vi "read numarray, compare with original one.vi"(0 "JSON in":string, 1 "binary data in":u8[](array[numeric]), 5 "array as variant in":variant, 7 "numeric type":T1, 9 "kwarg_name":string, 11 "error in (no error)":errorcluster, 12 "dims":u8) -> (2 "current timepoint":dbl, 3 "numarray 1D":cdb[](array[numeric]), 4 "numarray 2D":cdb[][](array[numeric]), 6 "numarray 3D":cdb[][][](array[numeric]), 8 "type out":dbl, 10 "arrays are equal":bool, 13 "delta t (s)":dbl, 15 "error out":errorcluster)   [LabVIEW 2018, in "LV2Julia_core.lvlib"]
uses:
  LV2Julia_core.lvlib
  Numeric Types enum.ctl
  f90f2f60-c893-4d73-9894-bda48d86c5b6.vi
  1bcb8ed7-17cb-4152-8e47-ff7461b55bf4.vi
  05796eaf-ec06-43a6-a453-a404cbedcfeb.vi
  9b93abbe-6376-4f86-9348-90245d6e1835.vi
  760e0b37-cac3-4b4c-a236-19af47651068.vi
  729fa7d7-fd6d-49c0-b1c8-f0a08cd6f943.vi
  3b835e31-b93c-4e4c-9ac3-413a3184b071.vi
  5ec570e5-464f-4fa0-a09b-d89833ec3b5d.vi
  e2ab0a43-58c4-4b3b-8f56-301dfe696cbe.vi
  7bf60a27-5564-4d89-912b-dc8cfc55a1e3.vi
  6c204d97-3017-4fe4-991a-9f71cab6a49b.vi
  a9a31f31-ba5d-4a99-a09b-6ec61be075e6.vi
  2bab1b1a-04a3-4102-80c6-0860ef51feeb.vi
  f90f2f60-c893-4d73-9894-bda48d86c5b6.vi/32d88ae3-2c92-48bd-897b-7dd0343570a7.vi
  f90f2f60-c893-4d73-9894-bda48d86c5b6.vi/c53afe73-fc52-444d-a3d7-7d50831e1209.vi
  f90f2f60-c893-4d73-9894-bda48d86c5b6.vi/a66dcc77-dec5-41f4-a21e-acddf706e10f.vi
  f90f2f60-c893-4d73-9894-bda48d86c5b6.vi/4ba7e992-ac92-4a49-a2e7-98c2637664ea.vi
  1bcb8ed7-17cb-4152-8e47-ff7461b55bf4.vi/43da8a50-dff1-4339-a1c3-934883bf3cfa.vi
  1bcb8ed7-17cb-4152-8e47-ff7461b55bf4.vi/d0f3aec3-e539-46ad-9ed6-51bc67961256.vi
  1bcb8ed7-17cb-4152-8e47-ff7461b55bf4.vi/9e853403-19d2-43d7-8698-e40b975fe7e1.vi
  1bcb8ed7-17cb-4152-8e47-ff7461b55bf4.vi/e786b37f-7961-4d73-906c-7eb43609efd0.vi
  05796eaf-ec06-43a6-a453-a404cbedcfeb.vi/e1d72838-30cd-489b-8a44-cd7fcf5818b4.vi
  05796eaf-ec06-43a6-a453-a404cbedcfeb.vi/17980820-88c9-4418-a022-c645ed7312dc.vi
  05796eaf-ec06-43a6-a453-a404cbedcfeb.vi/41ee7d88-6397-4a7e-920a-8c7af2978bc3.vi
  05796eaf-ec06-43a6-a453-a404cbedcfeb.vi/82dbf2c0-5480-4f2b-a01b-b6af73a511fc.vi
  9b93abbe-6376-4f86-9348-90245d6e1835.vi/4ad5f33a-0790-406d-bfe1-08bba8267a66.vi
  9b93abbe-6376-4f86-9348-90245d6e1835.vi/c16bd300-9a14-44dd-a8e2-ac449f43e7b5.vi
  9b93abbe-6376-4f86-9348-90245d6e1835.vi/a0511438-dd98-4a92-986f-621a9f363a6a.vi
  9b93abbe-6376-4f86-9348-90245d6e1835.vi/c651fa37-4a64-4550-919d-369354992084.vi
  760e0b37-cac3-4b4c-a236-19af47651068.vi/09310928-e73b-456e-a29f-2af550aeed02.vi
  760e0b37-cac3-4b4c-a236-19af47651068.vi/082161be-e65e-418d-b5c3-addb765fb303.vi
  760e0b37-cac3-4b4c-a236-19af47651068.vi/948893fb-24fe-4050-867c-ffeb5abdf6bc.vi
  760e0b37-cac3-4b4c-a236-19af47651068.vi/9bc4b464-3baf-47a8-acda-6a3046ee8e10.vi
  729fa7d7-fd6d-49c0-b1c8-f0a08cd6f943.vi/4dc461b2-c442-4aea-8fe2-f79e850e50b6.vi
  729fa7d7-fd6d-49c0-b1c8-f0a08cd6f943.vi/f3471e8a-deba-4189-9c10-aa71fc9210b9.vi
  729fa7d7-fd6d-49c0-b1c8-f0a08cd6f943.vi/32030ce2-dff6-4f01-95b7-0827d636a462.vi
  729fa7d7-fd6d-49c0-b1c8-f0a08cd6f943.vi/c713e3f1-cad3-46f2-84b7-66f09a7e94ff.vi
  3b835e31-b93c-4e4c-9ac3-413a3184b071.vi/28cea966-c3ee-4471-b26a-6f175bc131ac.vi
  3b835e31-b93c-4e4c-9ac3-413a3184b071.vi/de96e9b0-be66-4c9e-9efc-c1f704469a1d.vi
  3b835e31-b93c-4e4c-9ac3-413a3184b071.vi/c00be31e-9a51-4a5a-83a6-45b490b9e683.vi
  3b835e31-b93c-4e4c-9ac3-413a3184b071.vi/ac6c025d-f474-4280-83b8-e9f6b8e68690.vi
  5ec570e5-464f-4fa0-a09b-d89833ec3b5d.vi/ca82bea4-4b91-4f8b-9f61-83a2a5577914.vi
  5ec570e5-464f-4fa0-a09b-d89833ec3b5d.vi/c4c3de46-0252-44a8-9010-5f8eb92ca105.vi
  5ec570e5-464f-4fa0-a09b-d89833ec3b5d.vi/e4886903-d285-4e62-8f40-eb3ebe842de4.vi
  5ec570e5-464f-4fa0-a09b-d89833ec3b5d.vi/fb6f816f-daa7-4e23-ba72-f885aa13bf06.vi
  e2ab0a43-58c4-4b3b-8f56-301dfe696cbe.vi/4e651908-bd94-4c47-b669-930f4933d222.vi
  e2ab0a43-58c4-4b3b-8f56-301dfe696cbe.vi/36ea2579-6193-4f32-b3f5-d90bd214050e.vi
  e2ab0a43-58c4-4b3b-8f56-301dfe696cbe.vi/95d4ced7-8003-4378-85ae-3062075d27bb.vi
  e2ab0a43-58c4-4b3b-8f56-301dfe696cbe.vi/454c1be2-9309-4afe-9153-ec44cf4b9f7f.vi
  7bf60a27-5564-4d89-912b-dc8cfc55a1e3.vi/8069382f-b1d8-4b8c-8509-eebfa9e45f70.vi
  7bf60a27-5564-4d89-912b-dc8cfc55a1e3.vi/5c067dbe-246b-42e9-9137-861b00fe523e.vi
  7bf60a27-5564-4d89-912b-dc8cfc55a1e3.vi/03b17b19-1ffb-46cc-8dc1-1c496a915e89.vi
  7bf60a27-5564-4d89-912b-dc8cfc55a1e3.vi/ff1d2745-87c4-4d1c-a2b2-b7403a7ffa6b.vi
  6c204d97-3017-4fe4-991a-9f71cab6a49b.vi/511987f6-22be-4a86-9c96-591c0cf4b1f3.vi
  6c204d97-3017-4fe4-991a-9f71cab6a49b.vi/adae4af8-5be0-46d9-9bf5-f45836a08497.vi
  6c204d97-3017-4fe4-991a-9f71cab6a49b.vi/d2148ece-0ea0-4357-a1fc-e7d4a362048d.vi
  6c204d97-3017-4fe4-991a-9f71cab6a49b.vi/6f8aa3a7-2847-4f47-821d-e6fe881f478f.vi
  a9a31f31-ba5d-4a99-a09b-6ec61be075e6.vi/7f017d05-d453-41ac-95c6-3d882b468b72.vi
  a9a31f31-ba5d-4a99-a09b-6ec61be075e6.vi/c15c3db5-a9cc-4003-815d-eb9106ad24ec.vi
  a9a31f31-ba5d-4a99-a09b-6ec61be075e6.vi/a885508d-4bd5-4e1e-83f8-5cf6cb2b745b.vi
  a9a31f31-ba5d-4a99-a09b-6ec61be075e6.vi/8481d5d4-7fad-4bda-b605-7e699fe4b182.vi
  2bab1b1a-04a3-4102-80c6-0860ef51feeb.vi/7b08f5e4-8a18-4af1-a7e0-c238231d1d10.vi
  2bab1b1a-04a3-4102-80c6-0860ef51feeb.vi/3f7e7226-141b-4536-8259-caf852be88c8.vi
  2bab1b1a-04a3-4102-80c6-0860ef51feeb.vi/af87eeda-3917-4993-94e0-ad766b0f68b3.vi
  2bab1b1a-04a3-4102-80c6-0860ef51feeb.vi/5c378cb5-9f43-45ec-a4e5-82801b736eef.vi
  f90f2f60-c893-4d73-9894-bda48d86c5b6.vi/32d88ae3-2c92-48bd-897b-7dd0343570a7.vi/0a4ba05e-7b47-49e8-b08b-5e3ce4a88961.vi
  f90f2f60-c893-4d73-9894-bda48d86c5b6.vi/32d88ae3-2c92-48bd-897b-7dd0343570a7.vi/f92d9013-3aed-4396-b4da-6ee44087ecf7.vi
  <vilib>/Utility/High Resolution Relative Seconds.vi
  1bcb8ed7-17cb-4152-8e47-ff7461b55bf4.vi/43da8a50-dff1-4339-a1c3-934883bf3cfa.vi/c3af297e-0525-4c94-bb72-6317302d0e32.vi
  1bcb8ed7-17cb-4152-8e47-ff7461b55bf4.vi/43da8a50-dff1-4339-a1c3-934883bf3cfa.vi/790e9c30-092d-4b53-97d1-e3feff226708.vi
  05796eaf-ec06-43a6-a453-a404cbedcfeb.vi/e1d72838-30cd-489b-8a44-cd7fcf5818b4.vi/8b740511-b487-49ba-a093-73fb020563e9.vi
  05796eaf-ec06-43a6-a453-a404cbedcfeb.vi/e1d72838-30cd-489b-8a44-cd7fcf5818b4.vi/b666fddd-2d2a-4a6a-98a8-bbf63f924d98.vi
  9b93abbe-6376-4f86-9348-90245d6e1835.vi/4ad5f33a-0790-406d-bfe1-08bba8267a66.vi/3bd22be2-5111-47a8-b71b-fdc81ca5e66d.vi
  9b93abbe-6376-4f86-9348-90245d6e1835.vi/4ad5f33a-0790-406d-bfe1-08bba8267a66.vi/d137af0b-6666-4026-9fd6-31d3aa0aab9b.vi
  760e0b37-cac3-4b4c-a236-19af47651068.vi/09310928-e73b-456e-a29f-2af550aeed02.vi/18a4ba93-198a-457f-9888-6d837bbfc651.vi
  760e0b37-cac3-4b4c-a236-19af47651068.vi/09310928-e73b-456e-a29f-2af550aeed02.vi/36143d04-fe42-450e-9f83-4a025640125d.vi
  729fa7d7-fd6d-49c0-b1c8-f0a08cd6f943.vi/4dc461b2-c442-4aea-8fe2-f79e850e50b6.vi/fe959cfa-cdc2-4ee5-ae2a-48f0cffbfa1d.vi
  729fa7d7-fd6d-49c0-b1c8-f0a08cd6f943.vi/4dc461b2-c442-4aea-8fe2-f79e850e50b6.vi/ab9f782e-4743-4028-a12f-54521fe09be9.vi
  3b835e31-b93c-4e4c-9ac3-413a3184b071.vi/28cea966-c3ee-4471-b26a-6f175bc131ac.vi/fa75c5fa-ea52-4b08-9e23-d910e41973ba.vi
  3b835e31-b93c-4e4c-9ac3-413a3184b071.vi/28cea966-c3ee-4471-b26a-6f175bc131ac.vi/dc710c15-fbeb-4efa-8e36-deb9513761c7.vi
  5ec570e5-464f-4fa0-a09b-d89833ec3b5d.vi/ca82bea4-4b91-4f8b-9f61-83a2a5577914.vi/efdfd97e-ed7a-4a77-aa35-30702437550d.vi
  5ec570e5-464f-4fa0-a09b-d89833ec3b5d.vi/ca82bea4-4b91-4f8b-9f61-83a2a5577914.vi/a77c526b-b8bd-4cb0-918b-2e230f2ee520.vi
  e2ab0a43-58c4-4b3b-8f56-301dfe696cbe.vi/4e651908-bd94-4c47-b669-930f4933d222.vi/b91b84ad-bd5a-4b24-a288-76c801183de0.vi
  e2ab0a43-58c4-4b3b-8f56-301dfe696cbe.vi/4e651908-bd94-4c47-b669-930f4933d222.vi/530e12e3-75c7-4620-9169-231035b41acf.vi
  7bf60a27-5564-4d89-912b-dc8cfc55a1e3.vi/8069382f-b1d8-4b8c-8509-eebfa9e45f70.vi/d10227d4-541a-4949-87c7-fab712e9dd6e.vi
  7bf60a27-5564-4d89-912b-dc8cfc55a1e3.vi/8069382f-b1d8-4b8c-8509-eebfa9e45f70.vi/67064e3c-c67d-4289-9c66-d6cbd4a4f971.vi
  6c204d97-3017-4fe4-991a-9f71cab6a49b.vi/511987f6-22be-4a86-9c96-591c0cf4b1f3.vi/62feb09c-8c22-4b36-b42f-72fa80ada96d.vi
  6c204d97-3017-4fe4-991a-9f71cab6a49b.vi/511987f6-22be-4a86-9c96-591c0cf4b1f3.vi/d5a85607-7128-40a4-b7f6-5dda01c47754.vi
  a9a31f31-ba5d-4a99-a09b-6ec61be075e6.vi/7f017d05-d453-41ac-95c6-3d882b468b72.vi/8e6ae722-1908-4282-8b2b-0d284dc8bb27.vi
  a9a31f31-ba5d-4a99-a09b-6ec61be075e6.vi/7f017d05-d453-41ac-95c6-3d882b468b72.vi/20088c15-55a1-425e-abe7-bddea6ffbbe0.vi
  2bab1b1a-04a3-4102-80c6-0860ef51feeb.vi/7b08f5e4-8a18-4af1-a7e0-c238231d1d10.vi/3903ba21-d146-41e1-a685-2faba56e88ee.vi
  2bab1b1a-04a3-4102-80c6-0860ef51feeb.vi/7b08f5e4-8a18-4af1-a7e0-c238231d1d10.vi/29afcb73-7f9f-4903-94dc-9b6aba9bf54a.vi
  f90f2f60-c893-4d73-9894-bda48d86c5b6.vi/32d88ae3-2c92-48bd-897b-7dd0343570a7.vi/0a4ba05e-7b47-49e8-b08b-5e3ce4a88961.vi/efa4f8de-959a-4522-9046-8bf7e721ad25.vi
  1bcb8ed7-17cb-4152-8e47-ff7461b55bf4.vi/43da8a50-dff1-4339-a1c3-934883bf3cfa.vi/c3af297e-0525-4c94-bb72-6317302d0e32.vi/c9f4e11a-ed49-4902-bd07-aee6172cd663.vi
  05796eaf-ec06-43a6-a453-a404cbedcfeb.vi/e1d72838-30cd-489b-8a44-cd7fcf5818b4.vi/8b740511-b487-49ba-a093-73fb020563e9.vi/12a76261-bc90-4ade-a8aa-7cb656f356e6.vi
  9b93abbe-6376-4f86-9348-90245d6e1835.vi/4ad5f33a-0790-406d-bfe1-08bba8267a66.vi/3bd22be2-5111-47a8-b71b-fdc81ca5e66d.vi/a8d10c4b-4fce-4b82-b949-5b003fcb0e0a.vi
  760e0b37-cac3-4b4c-a236-19af47651068.vi/09310928-e73b-456e-a29f-2af550aeed02.vi/18a4ba93-198a-457f-9888-6d837bbfc651.vi/6730ac0e-5447-4b19-b35e-556b94703463.vi
  729fa7d7-fd6d-49c0-b1c8-f0a08cd6f943.vi/4dc461b2-c442-4aea-8fe2-f79e850e50b6.vi/fe959cfa-cdc2-4ee5-ae2a-48f0cffbfa1d.vi/3da4302c-71e9-4b31-b309-13f37399564a.vi
  3b835e31-b93c-4e4c-9ac3-413a3184b071.vi/28cea966-c3ee-4471-b26a-6f175bc131ac.vi/fa75c5fa-ea52-4b08-9e23-d910e41973ba.vi/fc83a91d-5b5c-4ecc-b21d-cf8973c7dde3.vi
  5ec570e5-464f-4fa0-a09b-d89833ec3b5d.vi/ca82bea4-4b91-4f8b-9f61-83a2a5577914.vi/efdfd97e-ed7a-4a77-aa35-30702437550d.vi/39ccba34-03b8-4678-b571-5cce52e08443.vi
  e2ab0a43-58c4-4b3b-8f56-301dfe696cbe.vi/4e651908-bd94-4c47-b669-930f4933d222.vi/b91b84ad-bd5a-4b24-a288-76c801183de0.vi/9d1a48f9-1ea6-42d2-9625-be3569ee797d.vi
  7bf60a27-5564-4d89-912b-dc8cfc55a1e3.vi/8069382f-b1d8-4b8c-8509-eebfa9e45f70.vi/d10227d4-541a-4949-87c7-fab712e9dd6e.vi/33778f74-64df-4093-b5dd-9a40335341ff.vi
  6c204d97-3017-4fe4-991a-9f71cab6a49b.vi/511987f6-22be-4a86-9c96-591c0cf4b1f3.vi/62feb09c-8c22-4b36-b42f-72fa80ada96d.vi/b7e7f7e1-f3ad-4205-8c28-679fe1259f1d.vi
  a9a31f31-ba5d-4a99-a09b-6ec61be075e6.vi/7f017d05-d453-41ac-95c6-3d882b468b72.vi/8e6ae722-1908-4282-8b2b-0d284dc8bb27.vi/c79da9b5-a081-427b-a98b-15fef315557e.vi
  <vilib>/Utility/error.llb/Error Cluster From Error Code.vi
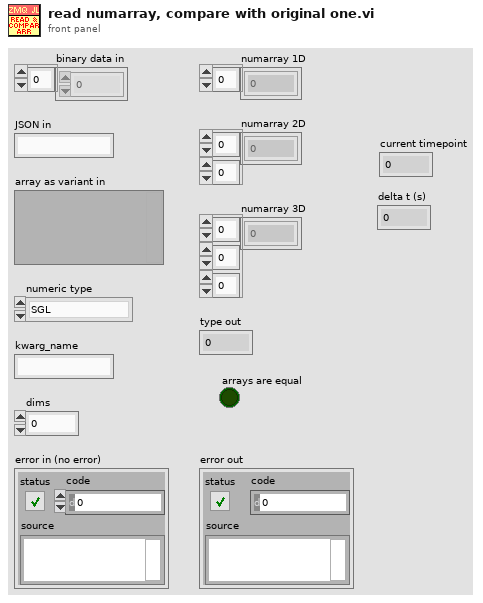
[diagram p1: front panel]
types:
  T1 = typedef "LV2Julia_core.lvlib/Numeric Types enum.ctl" = enum16{"SGL", "DBL", "I8", "I16", "I32", "I64", "U8", "U16", "U32", "U64", "CSGL", "CDBL", "boolean"}
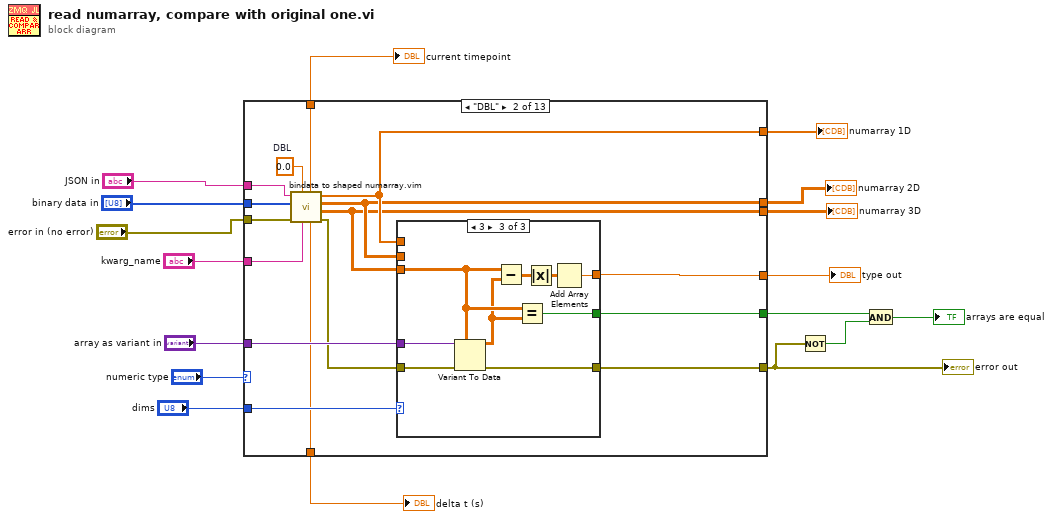
[diagram p0: block diagram]
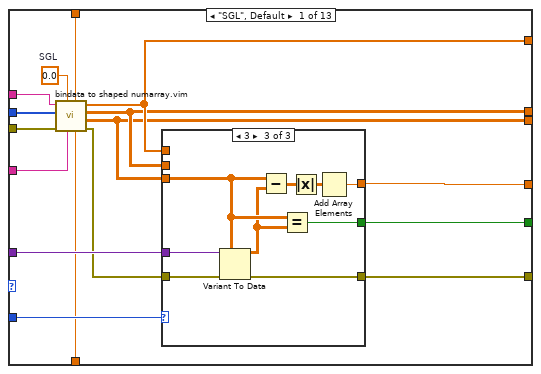
[diagram p2: hidden frame]
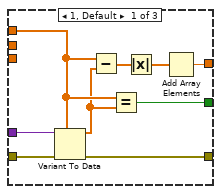
[diagram p3: hidden frame]
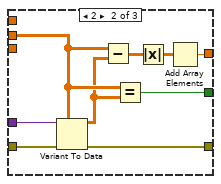
[diagram p4: hidden frame]
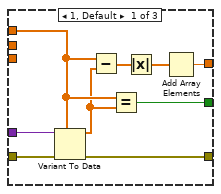
[diagram p5: hidden frame]
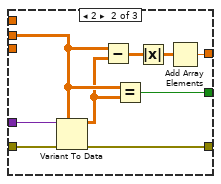
[diagram p6: hidden frame]
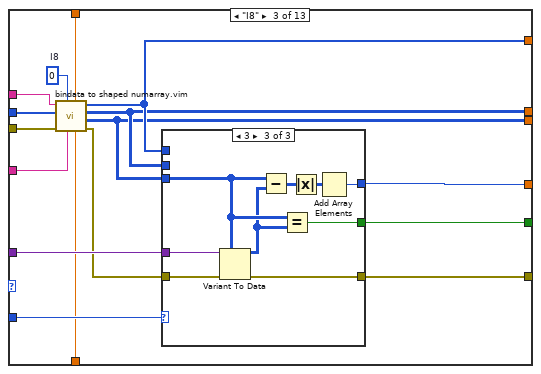
[diagram p7: hidden frame]
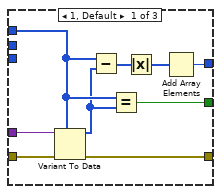
[diagram p8: hidden frame]
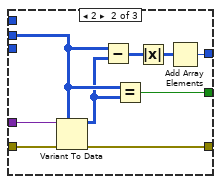
[diagram p9: hidden frame]
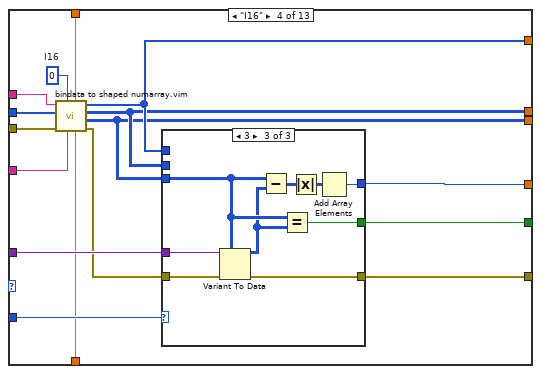
[diagram p10: hidden frame]
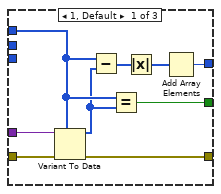
[diagram p11: hidden frame]
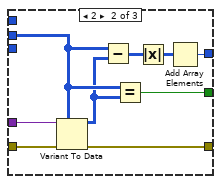
[diagram p12: hidden frame]
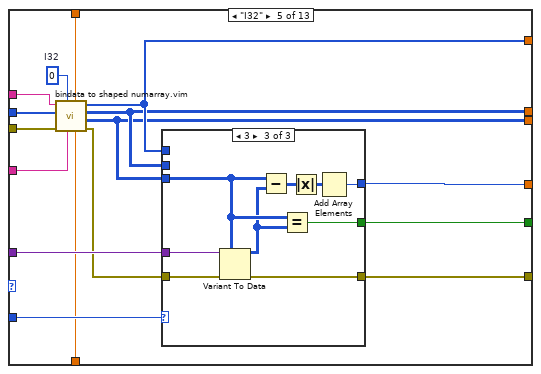
[diagram p13: hidden frame]
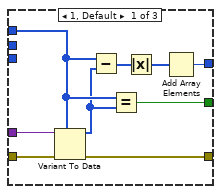
[diagram p14: hidden frame]
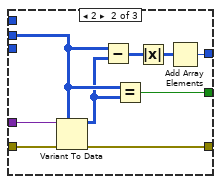
[diagram p15: hidden frame]
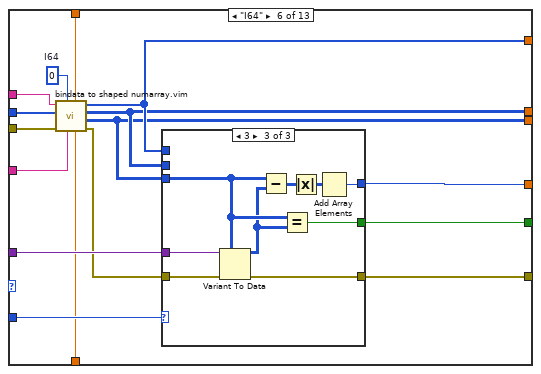
[diagram p16: hidden frame]
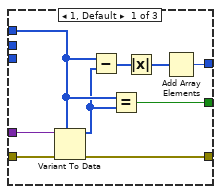
[diagram p17: hidden frame]
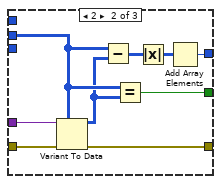
[diagram p18: hidden frame]
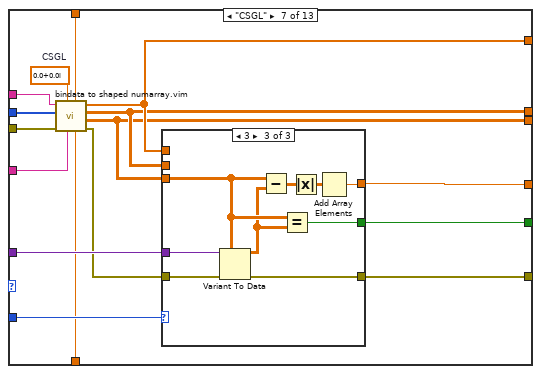
[diagram p19: hidden frame]
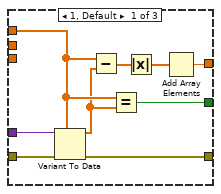
[diagram p20: hidden frame]
diagram:
  n1 = case shown="\"DBL\"" "numeric type" {
    tunnel: "error in (no error)" -> [w33 w76 w119 w162 w205 w248 w291 w334 w377 w417 w457 w497 w537]
    tunnel: "kwarg_name" -> [w32 w75 w118 w161 w204 w247 w290 w333 w376 w416 w456 w496 w536]
    tunnel: "binary data in" -> [w21 w63 w107 w150 w193 w236 w279 w322 w365 w405 w445 w485 w525]
    tunnel: "JSON in" -> [w20 w64 w106 w149 w192 w235 w278 w321 w364 w404 w444 w484 w524]
    tunnel: "dims" -> [w31 w74 w117 w160 w203 w246 w289 w332 w375 w415 w455 w495 w535]
    tunnel: [w30 w73 w116 w159 w202 w245 w288 w331 w374 w414 w454 w494 w534] -> w9
    tunnel: [w29 w72 w115 w158 w201 w244 w287 w330 w373 w413 w453 w493 w533] -> w10
    tunnel: [w28 w71 w114 w157 w200 w243 w286 w329 w372 w412 w452 w492 w532] -> w11
    tunnel: "array as variant in" -> [w27 w70 w113 w156 w199 w242 w285 w328 w371 w411 w451 w491 w531]
    tunnel: [w26 w69 w112 w155 w198 w241 w284 w327 w370 w410 w450 w490 w530] -> w4
    tunnel: [w25 w68 w111 w154 w197 w240 w283 w326 w369 w409 w449 w489 w529] -> w13
    tunnel: [w22 w65 w108 w151 w194 w237 w280 w323 w366 w406 w446 w486 w527] -> w14
    tunnel: [w19 w62 w105 w148 w191 w234 w277 w320 w363 w403 w443 w483 w523] -> w1
    tunnel: [w18 w61 w104 w147 w190 w233 w276 w319 w362 w402 w442 w482 w522] -> w2
    frame "SGL", Default {
      w23 = sgl 0.0  # SGL
      n2 = call "bindata to shaped numarray.vim"("name"=w32, "element type"=w23, "error in (no error)"=w33, "binary data"=w21, "JSON in"=w20) -> ("error out"=w24:errorcluster, "numarray 3D"=w25:sgl[][][], "numarray 2D"=w29:sgl[][], "numarray 1D"=w30:sgl[], "delta t (s)"=w18:dbl, "current timepoint"=w19:dbl)  [unwired: 1 in]
      n3 = case shown="3" w31 {
        tunnel: w30 -> [w36 _ _]
        tunnel: [w40 w49 w58] -> w28
        tunnel: w29 -> [_ w45 _]
        tunnel: w27 -> [w39 w48 w57]
        tunnel: w24 -> [w38 w47 w56]
        tunnel: [w37 w46 w55] -> w26
        tunnel: w25 -> [_ _ w54]
        tunnel: [w34 w43 w52] -> w22
        frame 1, Default {
          n4 = Variant To Data(error in=w38, type=w36, Variant=w39) -> (data=w35:sgl[], error out=w37:errorcluster)
          n5 = Subtract(x=w36, y=w35) -> (x-y=w42:sgl[])
          n6 = Equal?(x=w36, y=w35) -> (x = y?=w34:bool)
          n7 = Absolute Value(x=w42) -> (abs(x)=w41:sgl[])
          n8 = Add Array Elements(numeric array=w41) -> (sum=w40:sgl)
        }
        frame 2 {
          n9 = Variant To Data(error in=w47, type=w45, Variant=w48) -> (data=w44:sgl[][], error out=w46:errorcluster)
          n10 = Subtract(x=w45, y=w44) -> (x-y=w51:sgl[][])
          n11 = Equal?(x=w45, y=w44) -> (x = y?=w43:bool)
          n12 = Absolute Value(x=w51) -> (abs(x)=w50:sgl[][])
          n13 = Add Array Elements(numeric array=w50) -> (sum=w49:sgl)
        }
        frame 3 {
          n14 = Variant To Data(error in=w56, type=w54, Variant=w57) -> (data=w53:sgl[][][], error out=w55:errorcluster)
          n15 = Subtract(x=w54, y=w53) -> (x-y=w60:sgl[][][])
          n16 = Equal?(x=w54, y=w53) -> (x = y?=w52:bool)
          n17 = Absolute Value(x=w60) -> (abs(x)=w59:sgl[][][])
          n18 = Add Array Elements(numeric array=w59) -> (sum=w58:sgl)
        }
      }
    }
    frame "DBL" {
      w66 = 0.0  # DBL
      n19 = call "bindata to shaped numarray.vim"("name"=w75, "element type"=w66, "error in (no error)"=w76, "binary data"=w63, "JSON in"=w64) -> ("error out"=w67:errorcluster, "numarray 3D"=w68:dbl[][][], "numarray 2D"=w72:dbl[][], "numarray 1D"=w73:dbl[], "delta t (s)"=w61:dbl, "current timepoint"=w62:dbl)  [unwired: 1 in]
      n20 = case shown="3" w74 {
        tunnel: w73 -> [w79 _ _]
        tunnel: [w83 w92 w101] -> w71
        tunnel: w72 -> [_ w88 _]
        tunnel: w70 -> [w82 w91 w100]
        tunnel: w67 -> [w81 w90 w99]
        tunnel: [w80 w89 w98] -> w69
        tunnel: w68 -> [_ _ w97]
        tunnel: [w77 w86 w95] -> w65
        frame 1, Default {
          n21 = Variant To Data(error in=w81, type=w79, Variant=w82) -> (data=w78:dbl[], error out=w80:errorcluster)
          n22 = Subtract(x=w79, y=w78) -> (x-y=w85:dbl[])
          n23 = Equal?(x=w79, y=w78) -> (x = y?=w77:bool)
          n24 = Absolute Value(x=w85) -> (abs(x)=w84:dbl[])
          n25 = Add Array Elements(numeric array=w84) -> (sum=w83:dbl)
        }
        frame 2 {
          n26 = Variant To Data(error in=w90, type=w88, Variant=w91) -> (data=w87:dbl[][], error out=w89:errorcluster)
          n27 = Subtract(x=w88, y=w87) -> (x-y=w94:dbl[][])
          n28 = Equal?(x=w88, y=w87) -> (x = y?=w86:bool)
          n29 = Absolute Value(x=w94) -> (abs(x)=w93:dbl[][])
          n30 = Add Array Elements(numeric array=w93) -> (sum=w92:dbl)
        }
        frame 3 {
          n31 = Variant To Data(error in=w99, type=w97, Variant=w100) -> (data=w96:dbl[][][], error out=w98:errorcluster)
          n32 = Subtract(x=w97, y=w96) -> (x-y=w103:dbl[][][])
          n33 = Equal?(x=w97, y=w96) -> (x = y?=w95:bool)
          n34 = Absolute Value(x=w103) -> (abs(x)=w102:dbl[][][])
          n35 = Add Array Elements(numeric array=w102) -> (sum=w101:dbl)
        }
      }
    }
    frame "I8" {
      w109 = i8 0  # I8
      n36 = call "bindata to shaped numarray.vim"("name"=w118, "element type"=w109, "error in (no error)"=w119, "binary data"=w107, "JSON in"=w106) -> ("error out"=w110:errorcluster, "numarray 3D"=w111:i8[][][], "numarray 2D"=w115:i8[][], "numarray 1D"=w116:i8[], "delta t (s)"=w104:dbl, "current timepoint"=w105:dbl)  [unwired: 1 in]
      n37 = case shown="3" w117 {
        tunnel: w116 -> [w122 _ _]
        tunnel: [w126 w135 w144] -> w114
        tunnel: w115 -> [_ w131 _]
        tunnel: w113 -> [w125 w134 w143]
        tunnel: w110 -> [w124 w133 w142]
        tunnel: [w123 w132 w141] -> w112
        tunnel: w111 -> [_ _ w140]
        tunnel: [w120 w129 w138] -> w108
        frame 1, Default {
          n38 = Variant To Data(error in=w124, type=w122, Variant=w125) -> (data=w121:i8[], error out=w123:errorcluster)
          n39 = Subtract(x=w122, y=w121) -> (x-y=w128:i8[])
          n40 = Equal?(x=w122, y=w121) -> (x = y?=w120:bool)
          n41 = Absolute Value(x=w128) -> (abs(x)=w127:i8[])
          n42 = Add Array Elements(numeric array=w127) -> (sum=w126:i8)
        }
        frame 2 {
          n43 = Variant To Data(error in=w133, type=w131, Variant=w134) -> (data=w130:i8[][], error out=w132:errorcluster)
          n44 = Subtract(x=w131, y=w130) -> (x-y=w137:i8[][])
          n45 = Equal?(x=w131, y=w130) -> (x = y?=w129:bool)
          n46 = Absolute Value(x=w137) -> (abs(x)=w136:i8[][])
          n47 = Add Array Elements(numeric array=w136) -> (sum=w135:i8)
        }
        frame 3 {
          n48 = Variant To Data(error in=w142, type=w140, Variant=w143) -> (data=w139:i8[][][], error out=w141:errorcluster)
          n49 = Subtract(x=w140, y=w139) -> (x-y=w146:i8[][][])
          n50 = Equal?(x=w140, y=w139) -> (x = y?=w138:bool)
          n51 = Absolute Value(x=w146) -> (abs(x)=w145:i8[][][])
          n52 = Add Array Elements(numeric array=w145) -> (sum=w144:i8)
        }
      }
    }
    frame "I16" {
      w152 = i16 0  # I16
      n53 = call "bindata to shaped numarray.vim"("name"=w161, "element type"=w152, "error in (no error)"=w162, "binary data"=w150, "JSON in"=w149) -> ("error out"=w153:errorcluster, "numarray 3D"=w154:i16[][][], "numarray 2D"=w158:i16[][], "numarray 1D"=w159:i16[], "delta t (s)"=w147:dbl, "current timepoint"=w148:dbl)  [unwired: 1 in]
      n54 = case shown="3" w160 {
        tunnel: w159 -> [w165 _ _]
        tunnel: [w169 w178 w187] -> w157
        tunnel: w158 -> [_ w174 _]
        tunnel: w156 -> [w168 w177 w186]
        tunnel: w153 -> [w167 w176 w185]
        tunnel: [w166 w175 w184] -> w155
        tunnel: w154 -> [_ _ w183]
        tunnel: [w163 w172 w181] -> w151
        frame 1, Default {
          n55 = Variant To Data(error in=w167, type=w165, Variant=w168) -> (data=w164:i16[], error out=w166:errorcluster)
          n56 = Subtract(x=w165, y=w164) -> (x-y=w171:i16[])
          n57 = Equal?(x=w165, y=w164) -> (x = y?=w163:bool)
          n58 = Absolute Value(x=w171) -> (abs(x)=w170:i16[])
          n59 = Add Array Elements(numeric array=w170) -> (sum=w169:i16)
        }
        frame 2 {
          n60 = Variant To Data(error in=w176, type=w174, Variant=w177) -> (data=w173:i16[][], error out=w175:errorcluster)
          n61 = Subtract(x=w174, y=w173) -> (x-y=w180:i16[][])
          n62 = Equal?(x=w174, y=w173) -> (x = y?=w172:bool)
          n63 = Absolute Value(x=w180) -> (abs(x)=w179:i16[][])
          n64 = Add Array Elements(numeric array=w179) -> (sum=w178:i16)
        }
        frame 3 {
          n65 = Variant To Data(error in=w185, type=w183, Variant=w186) -> (data=w182:i16[][][], error out=w184:errorcluster)
          n66 = Subtract(x=w183, y=w182) -> (x-y=w189:i16[][][])
          n67 = Equal?(x=w183, y=w182) -> (x = y?=w181:bool)
          n68 = Absolute Value(x=w189) -> (abs(x)=w188:i16[][][])
          n69 = Add Array Elements(numeric array=w188) -> (sum=w187:i16)
        }
      }
    }
    frame "I32" {
      w195 = 0  # I32
      n70 = call "bindata to shaped numarray.vim"("name"=w204, "element type"=w195, "error in (no error)"=w205, "binary data"=w193, "JSON in"=w192) -> ("error out"=w196:errorcluster, "numarray 3D"=w197:i32[][][], "numarray 2D"=w201:i32[][], "numarray 1D"=w202:i32[], "delta t (s)"=w190:dbl, "current timepoint"=w191:dbl)  [unwired: 1 in]
      n71 = case shown="3" w203 {
        tunnel: w202 -> [w208 _ _]
        tunnel: [w212 w221 w230] -> w200
        tunnel: w201 -> [_ w217 _]
        tunnel: w199 -> [w211 w220 w229]
        tunnel: w196 -> [w210 w219 w228]
        tunnel: [w209 w218 w227] -> w198
        tunnel: w197 -> [_ _ w226]
        tunnel: [w206 w215 w224] -> w194
        frame 1, Default {
          n72 = Variant To Data(error in=w210, type=w208, Variant=w211) -> (data=w207:i32[], error out=w209:errorcluster)
          n73 = Subtract(x=w208, y=w207) -> (x-y=w214:i32[])
          n74 = Equal?(x=w208, y=w207) -> (x = y?=w206:bool)
          n75 = Absolute Value(x=w214) -> (abs(x)=w213:i32[])
          n76 = Add Array Elements(numeric array=w213) -> (sum=w212:i32)
        }
        frame 2 {
          n77 = Variant To Data(error in=w219, type=w217, Variant=w220) -> (data=w216:i32[][], error out=w218:errorcluster)
          n78 = Subtract(x=w217, y=w216) -> (x-y=w223:i32[][])
          n79 = Equal?(x=w217, y=w216) -> (x = y?=w215:bool)
          n80 = Absolute Value(x=w223) -> (abs(x)=w222:i32[][])
          n81 = Add Array Elements(numeric array=w222) -> (sum=w221:i32)
        }
        frame 3 {
          n82 = Variant To Data(error in=w228, type=w226, Variant=w229) -> (data=w225:i32[][][], error out=w227:errorcluster)
          n83 = Subtract(x=w226, y=w225) -> (x-y=w232:i32[][][])
          n84 = Equal?(x=w226, y=w225) -> (x = y?=w224:bool)
          n85 = Absolute Value(x=w232) -> (abs(x)=w231:i32[][][])
          n86 = Add Array Elements(numeric array=w231) -> (sum=w230:i32)
        }
      }
    }
    frame "I64" {
      w238 = i64 0  # I64
      n87 = call "bindata to shaped numarray.vim"("name"=w247, "element type"=w238, "error in (no error)"=w248, "binary data"=w236, "JSON in"=w235) -> ("error out"=w239:errorcluster, "numarray 3D"=w240:i64[][][], "numarray 2D"=w244:i64[][], "numarray 1D"=w245:i64[], "delta t (s)"=w233:dbl, "current timepoint"=w234:dbl)  [unwired: 1 in]
      n88 = case shown="3" w246 {
        tunnel: w245 -> [w251 _ _]
        tunnel: [w255 w264 w273] -> w243
        tunnel: w244 -> [_ w260 _]
        tunnel: w242 -> [w254 w263 w272]
        tunnel: w239 -> [w253 w262 w271]
        tunnel: [w252 w261 w270] -> w241
        tunnel: w240 -> [_ _ w269]
        tunnel: [w249 w258 w267] -> w237
        frame 1, Default {
          n89 = Variant To Data(error in=w253, type=w251, Variant=w254) -> (data=w250:i64[], error out=w252:errorcluster)
          n90 = Subtract(x=w251, y=w250) -> (x-y=w257:i64[])
          n91 = Equal?(x=w251, y=w250) -> (x = y?=w249:bool)
          n92 = Absolute Value(x=w257) -> (abs(x)=w256:i64[])
          n93 = Add Array Elements(numeric array=w256) -> (sum=w255:i64)
        }
        frame 2 {
          n94 = Variant To Data(error in=w262, type=w260, Variant=w263) -> (data=w259:i64[][], error out=w261:errorcluster)
          n95 = Subtract(x=w260, y=w259) -> (x-y=w266:i64[][])
          n96 = Equal?(x=w260, y=w259) -> (x = y?=w258:bool)
          n97 = Absolute Value(x=w266) -> (abs(x)=w265:i64[][])
          n98 = Add Array Elements(numeric array=w265) -> (sum=w264:i64)
        }
        frame 3 {
          n99 = Variant To Data(error in=w271, type=w269, Variant=w272) -> (data=w268:i64[][][], error out=w270:errorcluster)
          n100 = Subtract(x=w269, y=w268) -> (x-y=w275:i64[][][])
          n101 = Equal?(x=w269, y=w268) -> (x = y?=w267:bool)
          n102 = Absolute Value(x=w275) -> (abs(x)=w274:i64[][][])
          n103 = Add Array Elements(numeric array=w274) -> (sum=w273:i64)
        }
      }
    }
    frame "CSGL" {
      w281 = csg 0.0+0.0i  # CSGL
      n104 = call "bindata to shaped numarray.vim"("name"=w290, "element type"=w281, "error in (no error)"=w291, "binary data"=w279, "JSON in"=w278) -> ("error out"=w282:errorcluster, "numarray 3D"=w283:csg[][][], "numarray 2D"=w287:csg[][], "numarray 1D"=w288:csg[], "delta t (s)"=w276:dbl, "current timepoint"=w277:dbl)  [unwired: 1 in]
      n105 = case shown="3" w289 {
        tunnel: w288 -> [w294 _ _]
        tunnel: [w298 w307 w316] -> w286
        tunnel: w287 -> [_ w303 _]
        tunnel: w285 -> [w297 w306 w315]
        tunnel: w282 -> [w296 w305 w314]
        tunnel: [w295 w304 w313] -> w284
        tunnel: w283 -> [_ _ w312]
        tunnel: [w292 w301 w310] -> w280
        frame 1, Default {
          n106 = Variant To Data(error in=w296, type=w294, Variant=w297) -> (data=w293:csg[], error out=w295:errorcluster)
          n107 = Subtract(x=w294, y=w293) -> (x-y=w300:csg[])
          n108 = Equal?(x=w294, y=w293) -> (x = y?=w292:bool)
          n109 = Absolute Value(x=w300) -> (abs(x)=w299:sgl[])
          n110 = Add Array Elements(numeric array=w299) -> (sum=w298:sgl)
        }
        frame 2 {
          n111 = Variant To Data(error in=w305, type=w303, Variant=w306) -> (data=w302:csg[][], error out=w304:errorcluster)
          n112 = Subtract(x=w303, y=w302) -> (x-y=w309:csg[][])
          n113 = Equal?(x=w303, y=w302) -> (x = y?=w301:bool)
          n114 = Absolute Value(x=w309) -> (abs(x)=w308:sgl[][])
          n115 = Add Array Elements(numeric array=w308) -> (sum=w307:sgl)
        }
        frame 3 {
          n116 = Variant To Data(error in=w314, type=w312, Variant=w315) -> (data=w311:csg[][][], error out=w313:errorcluster)
          n117 = Subtract(x=w312, y=w311) -> (x-y=w318:csg[][][])
          n118 = Equal?(x=w312, y=w311) -> (x = y?=w310:bool)
          n119 = Absolute Value(x=w318) -> (abs(x)=w317:sgl[][][])
          n120 = Add Array Elements(numeric array=w317) -> (sum=w316:sgl)
        }
      }
    }
    frame "CDBL" {
      w324 = cdb 0.0+0.0i  # CDBL
      n121 = call "bindata to shaped numarray.vim"("name"=w333, "element type"=w324, "error in (no error)"=w334, "binary data"=w322, "JSON in"=w321) -> ("error out"=w325:errorcluster, "numarray 3D"=w326:cdb[][][], "numarray 2D"=w330:cdb[][], "numarray 1D"=w331:cdb[], "delta t (s)"=w319:dbl, "current timepoint"=w320:dbl)  [unwired: 1 in]
      n122 = case shown="3" w332 {
        tunnel: w331 -> [w337 _ _]
        tunnel: [w341 w350 w359] -> w329
        tunnel: w330 -> [_ w346 _]
        tunnel: w328 -> [w340 w349 w358]
        tunnel: w325 -> [w339 w348 w357]
        tunnel: [w338 w347 w356] -> w327
        tunnel: w326 -> [_ _ w355]
        tunnel: [w335 w344 w353] -> w323
        frame 1, Default {
          n123 = Variant To Data(error in=w339, type=w337, Variant=w340) -> (data=w336:cdb[], error out=w338:errorcluster)
          n124 = Subtract(x=w337, y=w336) -> (x-y=w343:cdb[])
          n125 = Equal?(x=w337, y=w336) -> (x = y?=w335:bool)
          n126 = Absolute Value(x=w343) -> (abs(x)=w342:dbl[])
          n127 = Add Array Elements(numeric array=w342) -> (sum=w341:dbl)
        }
        frame 2 {
          n128 = Variant To Data(error in=w348, type=w346, Variant=w349) -> (data=w345:cdb[][], error out=w347:errorcluster)
          n129 = Subtract(x=w346, y=w345) -> (x-y=w352:cdb[][])
          n130 = Equal?(x=w346, y=w345) -> (x = y?=w344:bool)
          n131 = Absolute Value(x=w352) -> (abs(x)=w351:dbl[][])
          n132 = Add Array Elements(numeric array=w351) -> (sum=w350:dbl)
        }
        frame 3 {
          n133 = Variant To Data(error in=w357, type=w355, Variant=w358) -> (data=w354:cdb[][][], error out=w356:errorcluster)
          n134 = Subtract(x=w355, y=w354) -> (x-y=w361:cdb[][][])
          n135 = Equal?(x=w355, y=w354) -> (x = y?=w353:bool)
          n136 = Absolute Value(x=w361) -> (abs(x)=w360:dbl[][][])
          n137 = Add Array Elements(numeric array=w360) -> (sum=w359:dbl)
        }
      }
    }
    frame "U8" {
      w367 = u8 0  # U8
      n138 = call "bindata to shaped numarray.vim"("name"=w376, "element type"=w367, "error in (no error)"=w377, "binary data"=w365, "JSON in"=w364) -> ("error out"=w368:errorcluster, "numarray 3D"=w369:u8[][][], "numarray 2D"=w373:u8[][], "numarray 1D"=w374:u8[], "delta t (s)"=w362:dbl, "current timepoint"=w363:dbl)  [unwired: 1 in]
      n139 = case shown="2" w375 {
        tunnel: w374 -> [w381 _ _]
        tunnel: [w385 w393 w401] -> w372
        tunnel: w373 -> [_ w389 _]
        tunnel: w371 -> [w384 w392 w400]
        tunnel: w368 -> [w383 w391 w399]
        tunnel: [w382 w390 w398] -> w370
        tunnel: w369 -> [_ _ w397]
        tunnel: [w379 w387 w395] -> w366
        frame 1, Default {
          n140 = Variant To Data(error in=w383, type=w381, Variant=w384) -> (data=w380:u8[], error out=w382:errorcluster)
          n141 = Subtract(x=w381, y=w380) -> (x-y=w378:u8[])
          n142 = Equal?(x=w381, y=w380) -> (x = y?=w379:bool)
          n143 = Add Array Elements(numeric array=w378) -> (sum=w385:u8)
        }
        frame 2 {
          n144 = Variant To Data(error in=w391, type=w389, Variant=w392) -> (data=w388:u8[][], error out=w390:errorcluster)
          n145 = Subtract(x=w389, y=w388) -> (x-y=w386:u8[][])
          n146 = Equal?(x=w389, y=w388) -> (x = y?=w387:bool)
          n147 = Add Array Elements(numeric array=w386) -> (sum=w393:u8)
        }
        frame 3 {
          n148 = Variant To Data(error in=w399, type=w397, Variant=w400) -> (data=w396:u8[][][], error out=w398:errorcluster)
          n149 = Subtract(x=w397, y=w396) -> (x-y=w394:u8[][][])
          n150 = Equal?(x=w397, y=w396) -> (x = y?=w395:bool)
          n151 = Add Array Elements(numeric array=w394) -> (sum=w401:u8)
        }
      }
    }
    frame "U16" {
      w407 = u16 0  # U16
      n152 = call "bindata to shaped numarray.vim"("name"=w416, "element type"=w407, "error in (no error)"=w417, "binary data"=w405, "JSON in"=w404) -> ("error out"=w408:errorcluster, "numarray 3D"=w409:u16[][][], "numarray 2D"=w413:u16[][], "numarray 1D"=w414:u16[], "delta t (s)"=w402:dbl, "current timepoint"=w403:dbl)  [unwired: 1 in]
      n153 = case shown="2" w415 {
        tunnel: w414 -> [w421 _ _]
        tunnel: [w425 w433 w441] -> w412
        tunnel: w413 -> [_ w429 _]
        tunnel: w411 -> [w424 w432 w440]
        tunnel: w408 -> [w423 w431 w439]
        tunnel: [w422 w430 w438] -> w410
        tunnel: w409 -> [_ _ w437]
        tunnel: [w419 w427 w435] -> w406
        frame 1, Default {
          n154 = Variant To Data(error in=w423, type=w421, Variant=w424) -> (data=w420:u16[], error out=w422:errorcluster)
          n155 = Subtract(x=w421, y=w420) -> (x-y=w418:u16[])
          n156 = Equal?(x=w421, y=w420) -> (x = y?=w419:bool)
          n157 = Add Array Elements(numeric array=w418) -> (sum=w425:u16)
        }
        frame 2 {
          n158 = Variant To Data(error in=w431, type=w429, Variant=w432) -> (data=w428:u16[][], error out=w430:errorcluster)
          n159 = Subtract(x=w429, y=w428) -> (x-y=w426:u16[][])
          n160 = Equal?(x=w429, y=w428) -> (x = y?=w427:bool)
          n161 = Add Array Elements(numeric array=w426) -> (sum=w433:u16)
        }
        frame 3 {
          n162 = Variant To Data(error in=w439, type=w437, Variant=w440) -> (data=w436:u16[][][], error out=w438:errorcluster)
          n163 = Subtract(x=w437, y=w436) -> (x-y=w434:u16[][][])
          n164 = Equal?(x=w437, y=w436) -> (x = y?=w435:bool)
          n165 = Add Array Elements(numeric array=w434) -> (sum=w441:u16)
        }
      }
    }
    frame "U32" {
      w447 = u32 0  # U32
      n166 = call "bindata to shaped numarray.vim"("name"=w456, "element type"=w447, "error in (no error)"=w457, "binary data"=w445, "JSON in"=w444) -> ("error out"=w448:errorcluster, "numarray 3D"=w449:u32[][][], "numarray 2D"=w453:u32[][], "numarray 1D"=w454:u32[], "delta t (s)"=w442:dbl, "current timepoint"=w443:dbl)  [unwired: 1 in]
      n167 = case shown="2" w455 {
        tunnel: w454 -> [w461 _ _]
        tunnel: [w465 w473 w481] -> w452
        tunnel: w453 -> [_ w469 _]
        tunnel: w451 -> [w464 w472 w480]
        tunnel: w448 -> [w463 w471 w479]
        tunnel: [w462 w470 w478] -> w450
        tunnel: w449 -> [_ _ w477]
        tunnel: [w459 w467 w475] -> w446
        frame 1, Default {
          n168 = Variant To Data(error in=w463, type=w461, Variant=w464) -> (data=w460:u32[], error out=w462:errorcluster)
          n169 = Subtract(x=w461, y=w460) -> (x-y=w458:u32[])
          n170 = Equal?(x=w461, y=w460) -> (x = y?=w459:bool)
          n171 = Add Array Elements(numeric array=w458) -> (sum=w465:u32)
        }
        frame 2 {
          n172 = Variant To Data(error in=w471, type=w469, Variant=w472) -> (data=w468:u32[][], error out=w470:errorcluster)
          n173 = Subtract(x=w469, y=w468) -> (x-y=w466:u32[][])
          n174 = Equal?(x=w469, y=w468) -> (x = y?=w467:bool)
          n175 = Add Array Elements(numeric array=w466) -> (sum=w473:u32)
        }
        frame 3 {
          n176 = Variant To Data(error in=w479, type=w477, Variant=w480) -> (data=w476:u32[][][], error out=w478:errorcluster)
          n177 = Subtract(x=w477, y=w476) -> (x-y=w474:u32[][][])
          n178 = Equal?(x=w477, y=w476) -> (x = y?=w475:bool)
          n179 = Add Array Elements(numeric array=w474) -> (sum=w481:u32)
        }
      }
    }
    frame "U64" {
      w487 = u64 0  # U64
      n180 = call "bindata to shaped numarray.vim"("name"=w496, "element type"=w487, "error in (no error)"=w497, "binary data"=w485, "JSON in"=w484) -> ("error out"=w488:errorcluster, "numarray 3D"=w489:u64[][][], "numarray 2D"=w493:u64[][], "numarray 1D"=w494:u64[], "delta t (s)"=w482:dbl, "current timepoint"=w483:dbl)  [unwired: 1 in]
      n181 = case shown="2" w495 {
        tunnel: w494 -> [w501 _ _]
        tunnel: [w505 w513 w521] -> w492
        tunnel: w493 -> [_ w509 _]
        tunnel: w491 -> [w504 w512 w520]
        tunnel: w488 -> [w503 w511 w519]
        tunnel: [w502 w510 w518] -> w490
        tunnel: w489 -> [_ _ w517]
        tunnel: [w499 w507 w515] -> w486
        frame 1, Default {
          n182 = Variant To Data(error in=w503, type=w501, Variant=w504) -> (data=w500:u64[], error out=w502:errorcluster)
          n183 = Subtract(x=w501, y=w500) -> (x-y=w498:u64[])
          n184 = Equal?(x=w501, y=w500) -> (x = y?=w499:bool)
          n185 = Add Array Elements(numeric array=w498) -> (sum=w505:u64)
        }
        frame 2 {
          n186 = Variant To Data(error in=w511, type=w509, Variant=w512) -> (data=w508:u64[][], error out=w510:errorcluster)
          n187 = Subtract(x=w509, y=w508) -> (x-y=w506:u64[][])
          n188 = Equal?(x=w509, y=w508) -> (x = y?=w507:bool)
          n189 = Add Array Elements(numeric array=w506) -> (sum=w513:u64)
        }
        frame 3 {
          n190 = Variant To Data(error in=w519, type=w517, Variant=w520) -> (data=w516:u64[][][], error out=w518:errorcluster)
          n191 = Subtract(x=w517, y=w516) -> (x-y=w514:u64[][][])
          n192 = Equal?(x=w517, y=w516) -> (x = y?=w515:bool)
          n193 = Add Array Elements(numeric array=w514) -> (sum=w521:u64)
        }
      }
    }
    frame "boolean" {
      n194 = call "bindata to shaped numarray.vim"("name"=w536, "element type"=TRUE, "error in (no error)"=w537, "binary data"=w525, "JSON in"=w524) -> ("error out"=w528:errorcluster, "numarray 3D"=w529:u8[][][], "numarray 2D"=w533:u8[][], "numarray 1D"=w534:u8[], "delta t (s)"=w522:dbl, "current timepoint"=w523:dbl)  [unwired: 1 in]
      n195 = case shown="3" w535 {
        tunnel: w534 -> [w538 _ _]
        tunnel: [w547 w557 w567] -> w532
        tunnel: w533 -> [_ w553 _]
        tunnel: w531 -> [w546 w556 w566]
        tunnel: w528 -> [w545 w555 w565]
        tunnel: [w544 w554 w564] -> w530
        tunnel: w529 -> [_ _ w558]
        tunnel: [w542 w551 w562] -> w527
        frame 1, Default {
          n196 = Variant To Data(error in=w545, type=bool[] [], Variant=w546) -> (data=w543:bool[], error out=w544:errorcluster)
          n197 = Boolean To (0,1)(Boolean=w543) -> (0, 1=w539:i16[])
          n198 = Subtract(x=w538, y=w539) -> (x-y=w541:i16[])
          n199 = Equal?(x=w538, y=w539) -> (x = y?=w542:bool)
          n200 = Add Array Elements(numeric array=w541) -> (sum=w547:i16)
        }
        frame 2 {
          n201 = Variant To Data(error in=w555, type=bool[][] [], Variant=w556) -> (data=w552:bool[][], error out=w554:errorcluster)
          n202 = Boolean To (0,1)(Boolean=w552) -> (0, 1=w548:i16[][])
          n203 = Subtract(x=w553, y=w548) -> (x-y=w550:i16[][])
          n204 = Equal?(x=w553, y=w548) -> (x = y?=w551:bool)
          n205 = Add Array Elements(numeric array=w550) -> (sum=w557:i16)
        }
        frame 3 {
          n206 = Variant To Data(error in=w565, type=bool[][][] [], Variant=w566) -> (data=w563:bool[][][], error out=w564:errorcluster)
          n207 = Boolean To (0,1)(Boolean=w563) -> (0, 1=w559:i16[][][])
          n208 = Subtract(x=w558, y=w559) -> (x-y=w561:i16[][][])
          n209 = Equal?(x=w558, y=w559) -> (x = y?=w562:bool)
          n210 = Add Array Elements(numeric array=w561) -> (sum=w567:i16)
        }
      }
    }
  }
  "numarray 3D" <- w13
  "error out" <- w4
  "type out" <- w11
  "numarray 2D" <- w10
  "numarray 1D" <- w9
  "delta t (s)" <- w2
  "current timepoint" <- w1
  n211 = Not(x=w4) -> (.not. x?=w3:bool)
  n212 = And(x=w14, y=w3) -> (x .and. y?=→"arrays are equal":bool)
